vi "获取固定格式的系统时间.vi"() -> (2 "毫秒计时值":u32, 3 "日期/时间字符串":string)   [LabVIEW 2015]
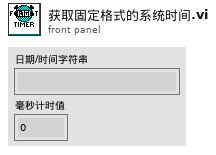
[diagram p1: front panel]
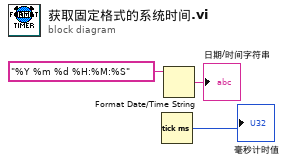
[diagram p0: block diagram]
diagram:
  n1 = Tick Count (ms)() -> (millisecond timer value=→"毫秒计时值":u32)
  n2 = Format Date/Time String(time format string (%c)="%Y %m %d %H:%M:%S" ("时间格式字符串(%c)")) -> (date/time string=→"日期/时间字符串":string)  [unwired: 2 in]
